vi "Write ACNET Devices to File.vi"(8 "error in (no error)":errorcluster, 10 "XML File Path":path, 11 "ACNET Devices in":refnum<class "ACNET Devices.lvclass">) -> (0 "error out":errorcluster, 3 "ACNET Devices out":refnum<class "ACNET Devices.lvclass">)   [LabVIEW 2013, in "ACNET Monitor.lvlib"]
uses:
  ACNET Devices.lvclass
  <vilib>/Utility/xml.llb/Write to XML File(string).vi
  ACNET Monitor.lvlib
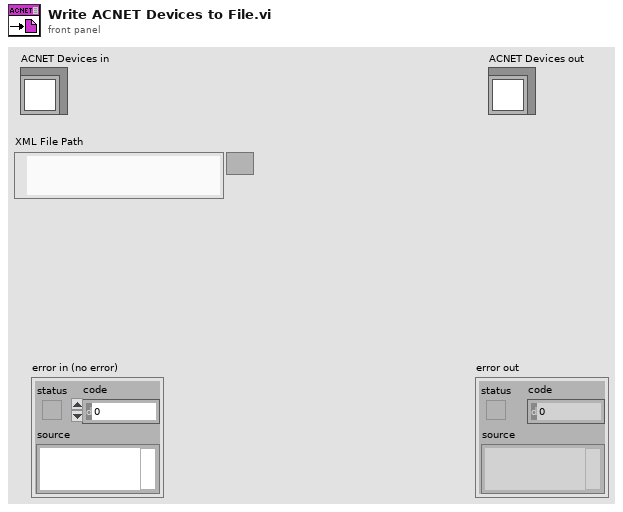
[diagram p1: front panel]
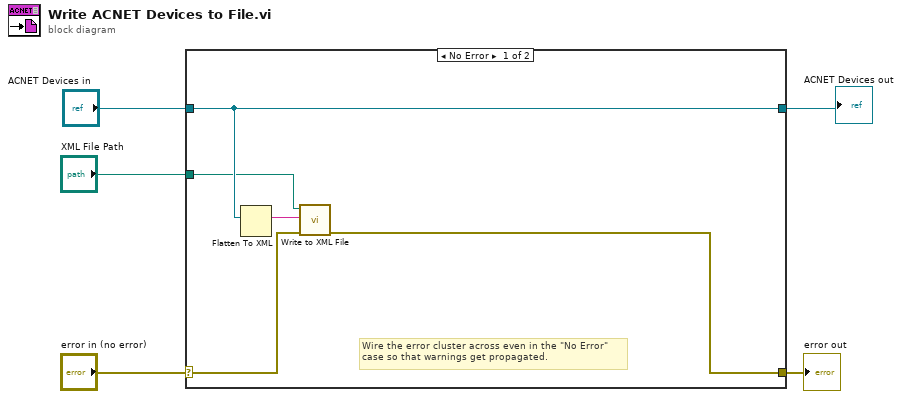
[diagram p0: block diagram]
diagram:
  n1 = case shown="No Error" "error in (no error)" {
    selector: "error in (no error)" -> [w7 w12]
    tunnel: [w6 w12] -> w4
    tunnel: [w9 w11] -> w1
    tunnel: "ACNET Devices in" -> [w9 w11]
    tunnel: "XML File Path" -> [w8 _]
    frame No Error {
      # "Wire the error cluster across even in the \"No Error\"\ncase so that warnings get propagated."
      n2 = Flatten To XML(anything=w9) -> (xml string=w10:string)
      n3 = call-poly <vilib>:"Write to XML File.vi"("error in (no error)"=w7, "XML Input"=w10, "XML File Path"=w8) -> ("error out"=w6:errorcluster)  [unwired: 6 in, 2 out]
    }
    frame Error {
    }
  }
  "error out" <- w4
  "ACNET Devices out" <- w1
